vi "VI Tree.vi"   [LabVIEW 2020, in "HandsOnPi2040.lvlib"]
doc: "This is the instrument driver for the <INSTRUMENT NAME>. The VI Tree displays all the user-callable VIs of the instrument driver in an organized table."
uses:
  <instrlib>/HandsOnPi2040/HandsOnPi2040.lvlib
panel:
  # "(c) 2014 <Enter Company Name Here>.  ALL RIGHTS RESERVED."
  # "SEE DIAGRAM\nFOR VI TREE."
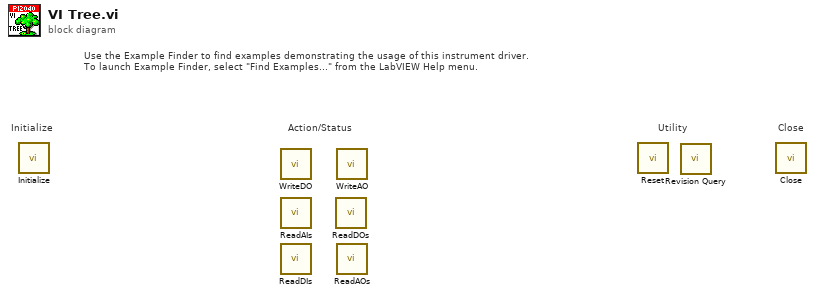
[diagram p0: block diagram]
diagram:
  # "Use the Example Finder to find examples demonstrating the usage of this instrument driver.\nTo launch Example Finder, select \"Find Examples...\" from the LabVIEW Help menu."
  # "Utility"
  # "Action/Status"
  # "Close"
  # "Initialize"
  n1 = call <instrlib>:"Initialize.vi"() -> ()  [unwired: 9 in, 3 out]
  n2 = call <instrlib>:"WriteDO.vi"() -> ()  [unwired: 10 in, 2 out]
  n3 = call <instrlib>:"ReadAIs.vi"() -> ()  [unwired: 9 in, 3 out]
  n4 = call <instrlib>:"ReadDIs.vi"() -> ()  [unwired: 9 in, 3 out]
  n5 = call <instrlib>:"ReadDOs.vi"() -> ()  [unwired: 9 in, 3 out]
  n6 = call <instrlib>:"WriteAO.vi"() -> ()  [unwired: 10 in, 2 out]
  n7 = call <instrlib>:"ReadAOs.vi"() -> ()  [unwired: 9 in, 3 out]
  n8 = call <instrlib>:"Reset.vi"() -> ()  [unwired: 10 in, 2 out]
  n9 = call <instrlib>:"Revision Query.vi"() -> ()  [unwired: 8 in, 4 out]
  n10 = call <instrlib>:"Close.vi"() -> ()  [unwired: 11 in, 1 out]
